vi "3Dv2.vi"(9 "Z-Position":dbl format="%#_13g") -> (0 "reference out":refnum<vi>)   [LabVIEW 2023]
uses:
  <vilib>/picture/3D Picture Control/Object/Create Object (name).vi
  <vilib>/picture/3D Picture Control/Object/Add Object (no reference).vi
  <vilib>/picture/3D Picture Control/NI_3D Picture Control.lvlib
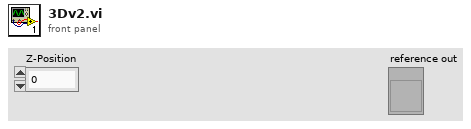
[diagram p1: front panel]
types:
  T1 = cluster{"Red":sgl, "Green":sgl, "Blue":sgl, "Alpha":sgl}
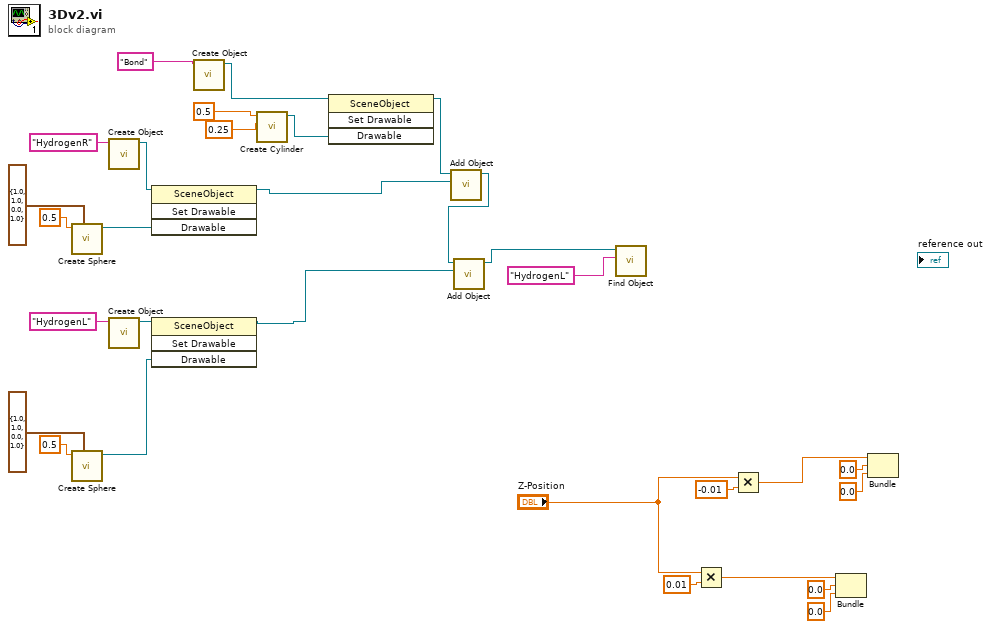
[diagram p0: block diagram]
diagram:
  n1 = call <vilib>:"Create Sphere.vi"("Color"=T1 {"Red"=1.0, "Green"=1.0, "Blue"=0.0, "Alpha"=1.0}, "Radius"=sgl 0.5) -> ("New Sphere Refnum"=w26:refnum<vi>)  [unwired: 8 in, 1 out]
  n2 = call <vilib>:"Create Sphere.vi"("Color"=T1 {"Red"=1.0, "Green"=1.0, "Blue"=0.0, "Alpha"=1.0}, "Radius"=sgl 0.5) -> ("New Sphere Refnum"=w21:refnum<vi>)  [unwired: 8 in, 1 out]
  n3 = call-poly <vilib>:"Create Object.vi"("Name"="HydrogenR") -> ("Scene:New Object"=w28:refnum<vi>)  [unwired: 9 in, 1 out]
  n4 = call-poly <vilib>:"Create Object.vi"("Name"="HydrogenL") -> ("Scene:New Object"=w23:refnum<vi>)  [unwired: 9 in, 1 out]
  n5 = invoke class="SceneObject" method="Set Drawable"(reference=w28, "Drawable"=w26) -> (reference out=w5:refnum<vi>)  [unwired: 2 in, 3 out]
  n6 = invoke class="SceneObject" method="Set Drawable"(reference=w23, "Drawable"=w21) -> (reference out=w4:refnum<vi>)  [unwired: 2 in, 3 out]
  n7 = call-poly <vilib>:"Create Object.vi"("Name"="Bond") -> ("Scene:New Object"=w10:refnum<vi>)  [unwired: 9 in, 1 out]
  n8 = call <vilib>:"Create Cylinder.vi"("Radius"=sgl 0.25, "Height"=sgl 0.5) -> ("New Cylinder Refnum"=w11:refnum<vi>)  [unwired: 8 in, 1 out]
  n9 = invoke class="SceneObject" method="Set Drawable"(reference=w10, "Drawable"=w11) -> (reference out=w3:refnum<vi>)  [unwired: 2 in, 3 out]
  n10 = call-poly <vilib>:"Add Object.vi"("New Object In"=w5, "Scene Object In"=w3) -> ("Scene Object Out"=w12:refnum<vi>)  [unwired: 8 in, 1 out]
  n11 = call-poly <vilib>:"Add Object.vi"("New Object In"=w4, "Scene Object In"=w12) -> ("Scene Object Out"=w2:refnum<vi>)  [unwired: 8 in, 1 out]
  n12 = call <vilib>:"Find Object.vi"("Object Name"="HydrogenL", "Scene Refnum"=w2) -> ()  [unwired: 8 in, 2 out]
  n13 = Multiply(x="Z-Position", y=0.01) -> (x*y=w6:dbl)
  n14 = Multiply(x="Z-Position", y=-0.01) -> (x*y=w13:dbl)
  n15 = Bundle(w6, 0.0, 0.0) -> ()  [unwired: 1 in, 1 out]
  n16 = Bundle(w13, 0.0, 0.0) -> ()  [unwired: 1 in, 1 out]
